vi "Analyzer.RequirementFileNameObtainer.vi"(0 "CSV Directory":path, 1 "Operation":enum16{"Reset", "Get"}(ring), 11 "error in":errorcluster) -> (4 "File Path":path, 6 "End of List":bool, 15 "error out":errorcluster)   [LabVIEW 2022 SP3, in "Analyzer.lvclass"]
uses:
  Analyzer.lvclass
  Analyzer.lvclass/Analyzer.ctl
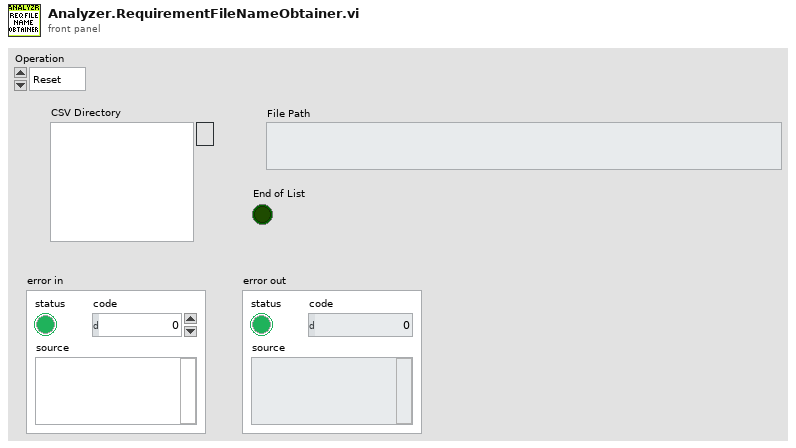
[diagram p1: front panel]
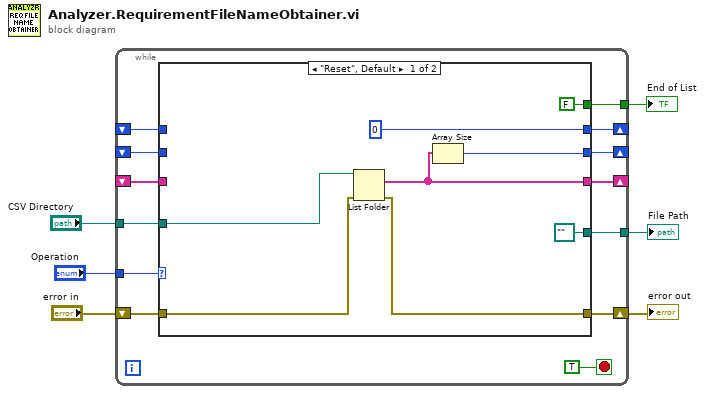
[diagram p0: block diagram]
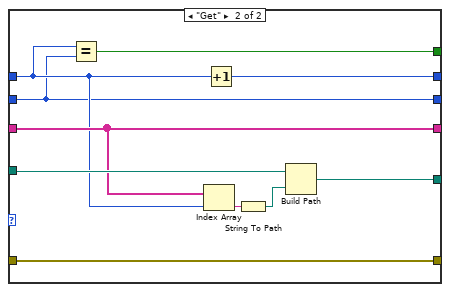
[diagram p2: hidden frame]
diagram:
  n1 = while {
    tunnel: "Operation" -> [w18]
    tunnel: "CSV Directory" -> [w17]
    shift-right: [w16] -> _
    shift-left: _ -> [w15]
    shift-right: [w14] -> _
    shift-left: _ -> [w13]
    shift-right: [w11] -> w3
    shift-left: "error in" -> [w12]
    tunnel: [w10] -> w2
    shift-right: [w9] -> _
    shift-left: _ -> [w8]
    tunnel: [w7] -> w1
    stop <- TRUE stop-if-true
    n2 = case shown="\"Reset\", Default" w18 {
      tunnel: w17 -> [w26 w36]
      tunnel: [0 w37] -> w16
      tunnel: w15 -> [_ w30]
      tunnel: [w22 w31] -> w14
      tunnel: w13 -> [_ w31]
      tunnel: w12 -> [w25 w32]
      tunnel: [w24 w32] -> w11
      tunnel: [path "" ("appended path") w33] -> w10
      tunnel: [w21 w28] -> w9
      tunnel: w8 -> [_ w28]
      tunnel: [FALSE w29] -> w7
      frame "Reset", Default {
        n3 = List Folder(path=w26, error in=w25) -> (filenames=w22:string[], error out=w24:errorcluster)  [unwired: 2 in, 2 out]
        n4 = Array Size(array=w22) -> (size(s)=w21:i32)
      }
      frame "Get" {
        n5 = Equal?(x=w30, y=w28) -> (x = y?=w29:bool)
        n6 = Index Array(array=w31, index=w30) -> (element=w35:string)
        n7 = Increment(x=w30) -> (x+1=w37:i32)
        n8 = String To Path(string=w35) -> (path=w34:path)
        n9 = Build Path(base path=w36, name or relative path=w34) -> (appended path=w33:path)
      }
    }
  }
  "File Path" <- w2
  "error out" <- w3
  "End of List" <- w1
